vi "CDR.vi"(4 "Mass Flow (kg/s)":dbl, 6 "Density (kg/m^3)":dbl, 7 "HX Power (W)":dbl, 8 "Cold Vol (m^3)":dbl=2.226 format="%#_13g", 9 "Cp (J/kgK)":dbl, 10 "Delta T (K)":dbl, 11 "Time (s)":dbl) -> (3 "Cooldown (K)":dbl)   [LabVIEW 2019]
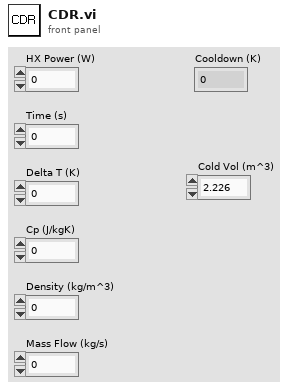
[diagram p1: front panel]
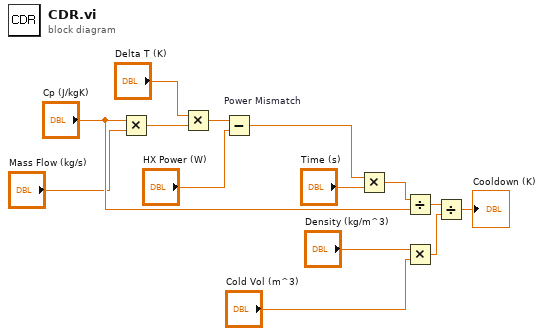
[diagram p0: block diagram]
diagram:
  n1 = Multiply(x="Cp (J/kgK)", y="Mass Flow (kg/s)") -> (x*y=w3:dbl)
  n2 = Multiply(x="Delta T (K)", y=w3) -> (x*y=w4:dbl)
  n3 = Subtract "Power Mismatch"(x=w4, y="HX Power (W)") -> (x-y=w7:dbl)
  n4 = Multiply(x=w7, y="Time (s)") -> (x*y=w8:dbl)
  n5 = Divide(x=w8, y="Cp (J/kgK)") -> (x/y=w13:dbl)
  n6 = Multiply(x="Density (kg/m^3)", y="Cold Vol (m^3)") -> (x*y=w12:dbl)
  n7 = Divide(x=w13, y=w12) -> (x/y=→"Cooldown (K)":dbl)
